vi "EMG.vi"() -> ()   [LabVIEW 2023]
uses:
  <vilib>/Analysis/3filter.llb/Butterworth Filter (DBL).vi
  <vilib>/Analysis/NI_AALBase.lvlib
panel:
  out "Waveform Graph 2":dbl[](graph)
  out "Waveform Graph":waveform(dbl)(graph)
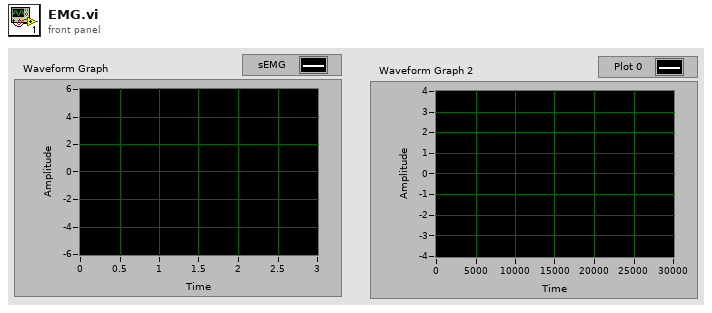
[diagram p1: front panel]
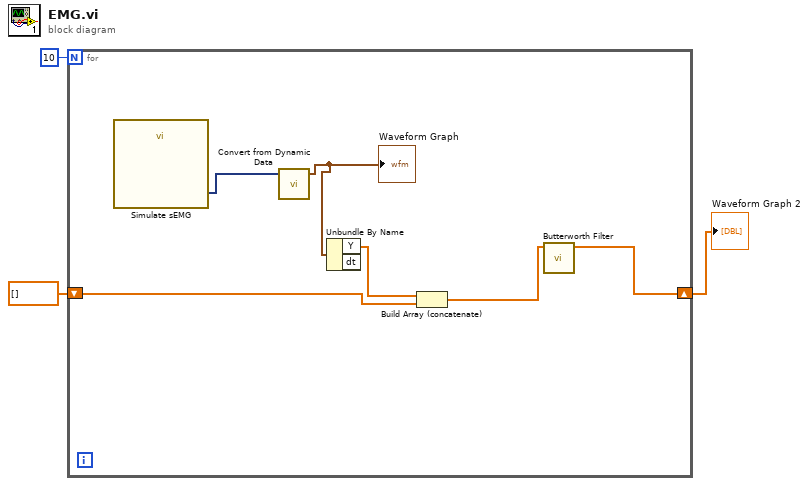
[diagram p0: block diagram]
diagram:
  n1 = for {
    N: 10 -> [_]
    shift-right: [w4] -> w3
    shift-left: dbl[] [] -> [w6]
    n2 = call "Simulate sEMG"() -> ("EMG"=w9:dynamicdata)  [unwired: 10 in, 1 out]
    n3 = call "Convert from Dynamic Data"("Dynamic Data Type"=w9) -> ("Waveform"=w8:waveform(dbl))  [unwired: 3 in]
    "Waveform Graph" <- w8
    n4 = Unbundle By Name(w8) -> ("Y"=w7:dbl[])  [unwired: 1 out]
    n5 = Build Array (concatenate)(w7, w6) -> (w5:dbl[])
    n6 = call-poly <vilib>:"Butterworth Filter.vi"("X"=w5) -> ("Filtered X"=w4:dbl[])  [unwired: 7 in, 1 out]
  }
  "Waveform Graph 2" <- w3
